vi "Set Ring Strings and Values.vi"   [LabVIEW 2020, in "Ring Field.lvclass"]
uses:
  Ring Field.lvclass
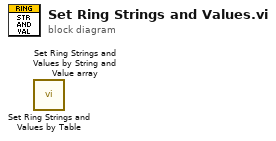
[diagram p0: block diagram]
diagram:
  n1 = call "Set Ring Strings and Values by Table.vi"() -> ()  [unwired: 10 in, 2 out]
  n2 = call "Set Ring Strings and Values by String and Value array.vi"() -> ()  [unwired: 10 in, 2 out]
